vi "RT Loop - Acquisition and Logging V2.vi"(8 "error in (no error)":errorcluster, 9 "Acquisition and Logging Configuration":T1={"Data Rate"=1, "Samples per Read"=0, "Number of Reads to Save"=0, "Data File Name"="", "TDMS Properties"=[], "Number of Channels"=4, "Channel Scale Array"=[0.0, 0.0, 0.0, 0.0, 1.0, 1.0, 1.0, 1.0], "Channel Names"=[], "Trigger - RMS Value"=0.0, "Trigger - Channel"=0, "Trigger - Time (Minute)"=0} {"Data Rate" items=["51.200 kS/s (NI 9234)"=1, "25.600 kS/s (NI 9234)"=2, "17.067 kS/s (NI 9234)"=3, "12.800 kS/s (NI 9234)"=4, "10.240 kS/s (NI 9234)"=5, "8.533 kS/s (NI 9234)"=6, "7.314 kS/s (NI 9234)"=7, "6.400 kS/s (NI 9234)"=8, "5.689 kS/s (NI 9234)"=9, "5.120 kS/s (NI 9234)"=10, "4.654 kS/s (NI 9234)"=11, "4.267 kS/s (NI 9234)"=12, "3.938 kS/s (NI 9234)"=13, "3.657 kS/s (NI 9234)"=14, "3.413 kS/s (NI 9234)"=15, "3.200 kS/s (NI 9234)"=16, "3.012 kS/s (NI 9234)"=17, "2.845 kS/s (NI 9234)"=18, "2.695 kS/s (NI 9234)"=19, "2.560 kS/s (NI 9234)"=20, "2.438 kS/s (NI 9234)"=21, "2.328 kS/s (NI 9234)"=22, "2.226 kS/s (NI 9234)"=23, "2.133 kS/s (NI 9234)"=24, "2.048 kS/s (NI 9234)"=25, "1.969 kS/s (NI 9234)"=26, "1.896 kS/s (NI 9234)"=27, "1.829 kS/s (NI 9234)"=28, "1.765 kS/s (NI 9234)"=29, "1.707 kS/s (NI 9234)"=30, "1.652 kS/s (NI 9234)"=31]}, 10 "Acquisition and Logging Queue":refnum<queue>, 11 "Message Queue":refnum<queue>) -> ()   [LabVIEW 2015]
uses:
  controls/FPGA VI Reference.ctl
  support/Message Queue/Message Queue.lvlib
  Globals/Global - Configuration Options.vi
  Globals/Global - Monitoring Variables.vi
  support/Message Queue/Message Cluster.ctl
  controls/Acquisition and Logging Configuration.ctl
  <vilib>/LabVIEW Targets/FPGA/cRIO/shared/nicrio_ModuleControls/nicrio_cRIO-9234_DataRatesRing2.ctl
  controls/TDMS Properties.ctl
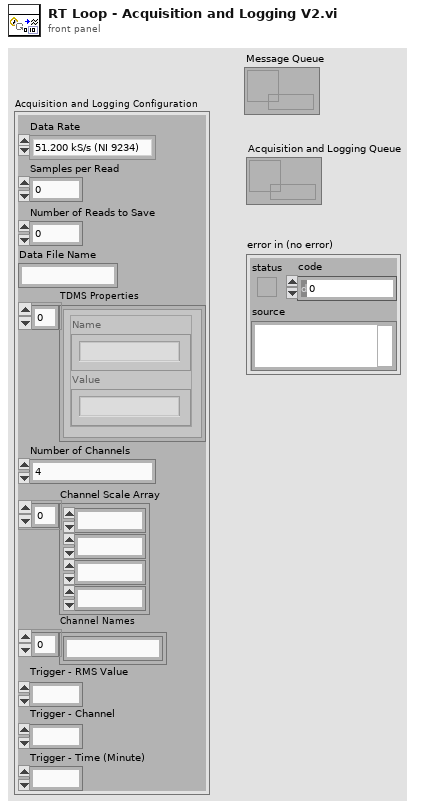
[diagram p1: front panel]
types:
  T1 = typedef "Acquisition and Logging Configuration.ctl" = cluster{"Data Rate":T2, "Samples per Read":i32, "Number of Reads to Save":i32, "Data File Name":string, "TDMS Properties":T3[], "Number of Channels":i32, "Channel Scale Array":fxp<+,24,12>[], "Channel Names":string[], "Trigger - RMS Value":dbl, "Trigger - Channel":i32, "Trigger - Time (Minute)":i32}
  T2 = typedef "nicrio_cRIO-9234_DataRatesRing2.ctl" = u8
  T3 = typedef "TDMS Properties.ctl" = cluster{"Name":string, "Value":string}
  T4 = typedef "FPGA VI Reference.ctl" = refnum<k20>
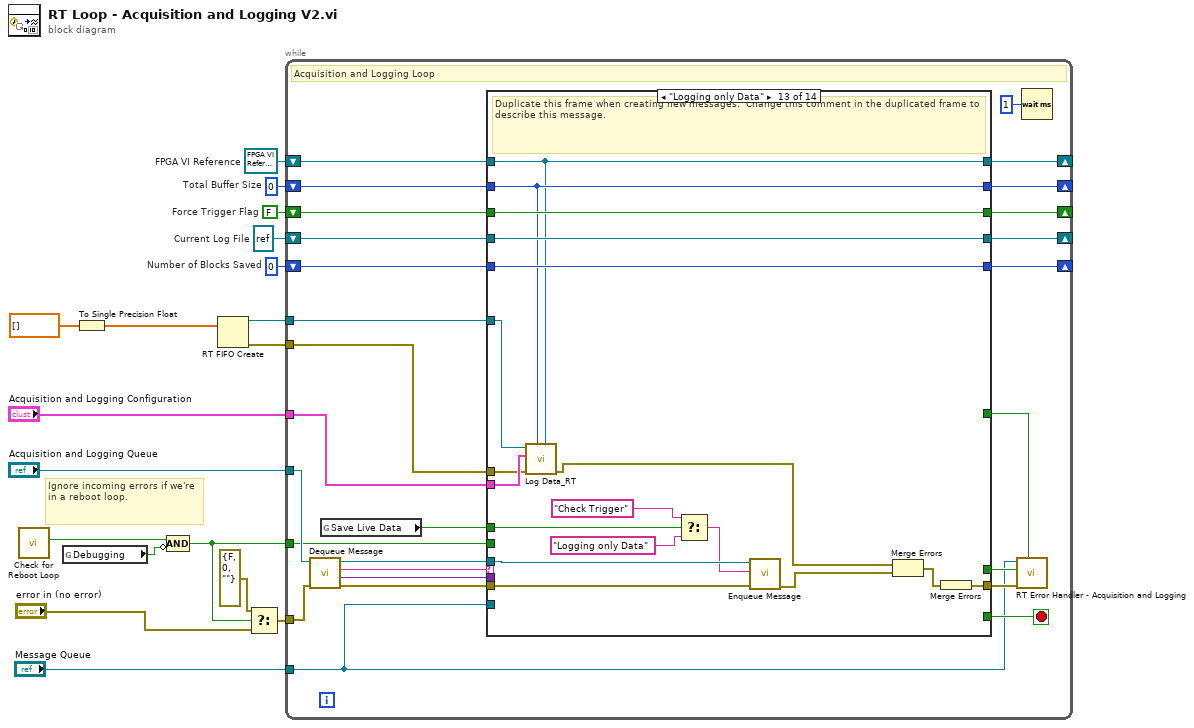
[diagram p0: block diagram]
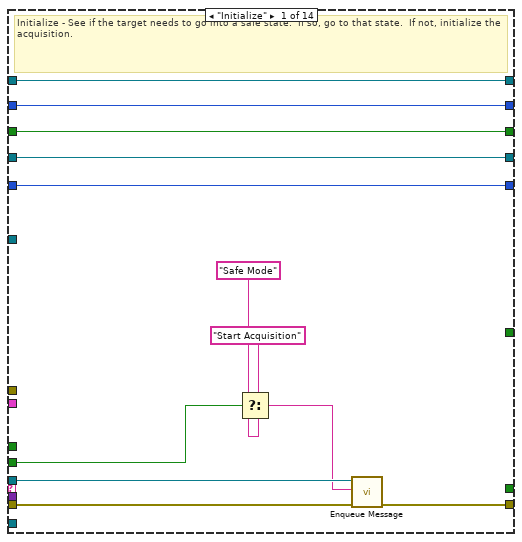
[diagram p2: hidden frame]
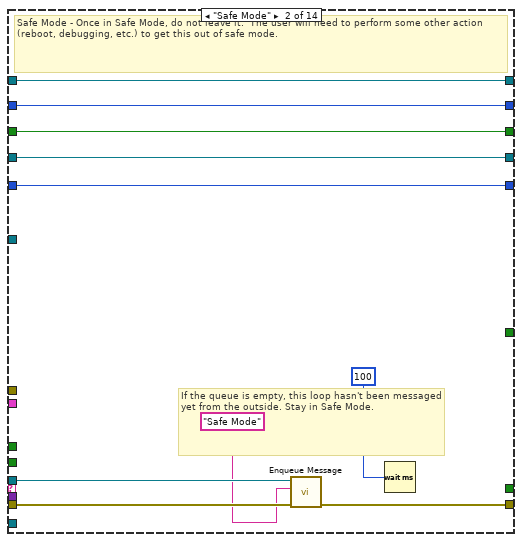
[diagram p3: hidden frame]
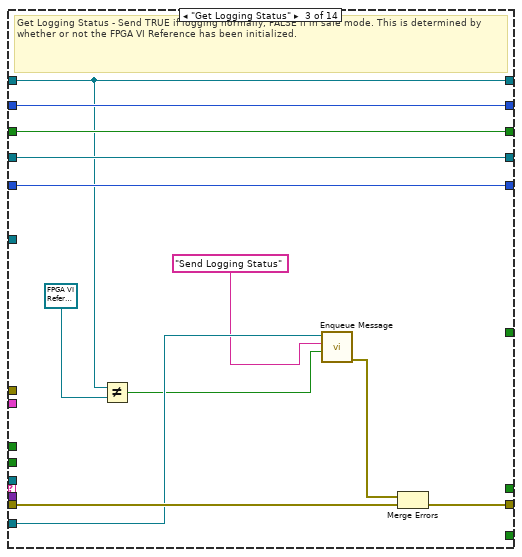
[diagram p4: hidden frame]
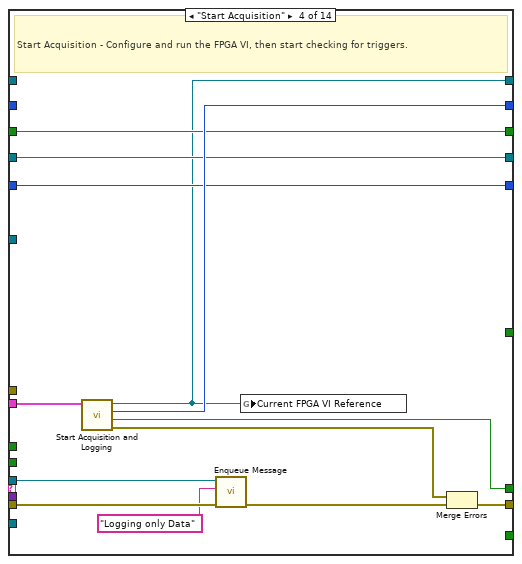
[diagram p5: hidden frame]
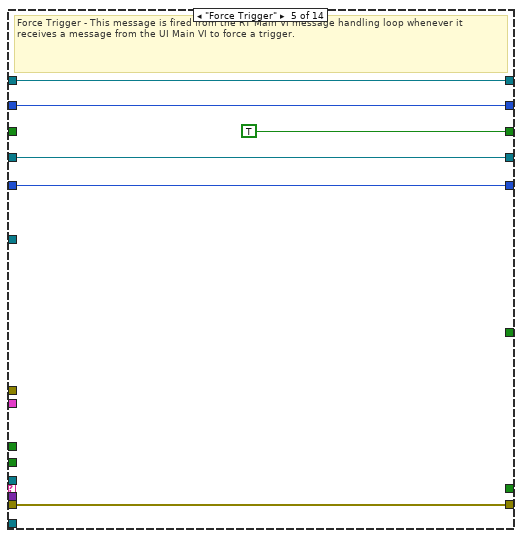
[diagram p6: hidden frame]
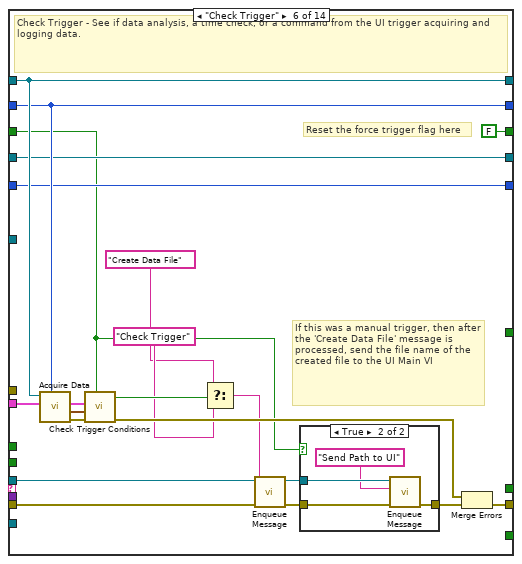
[diagram p7: hidden frame]
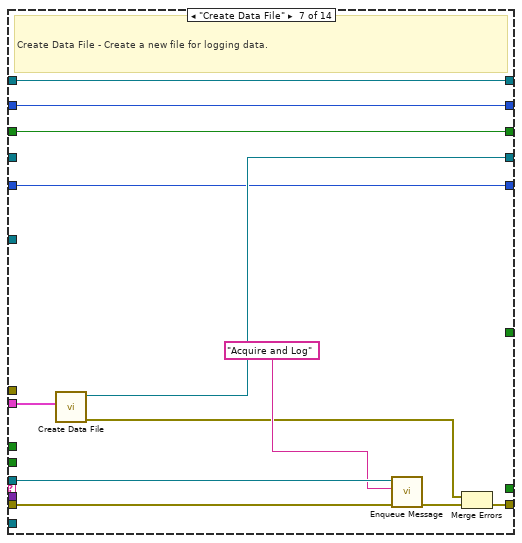
[diagram p9: hidden frame]
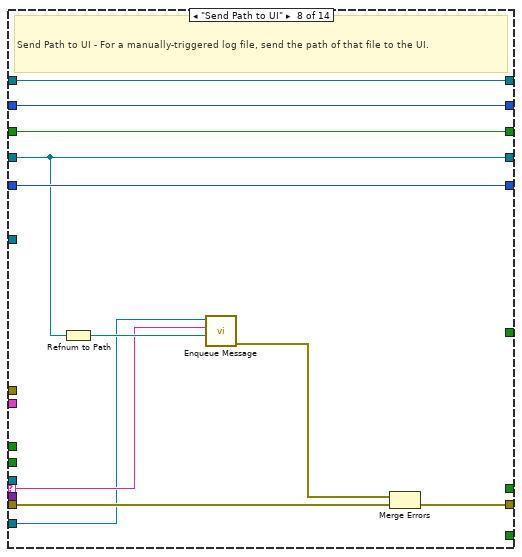
[diagram p10: hidden frame]
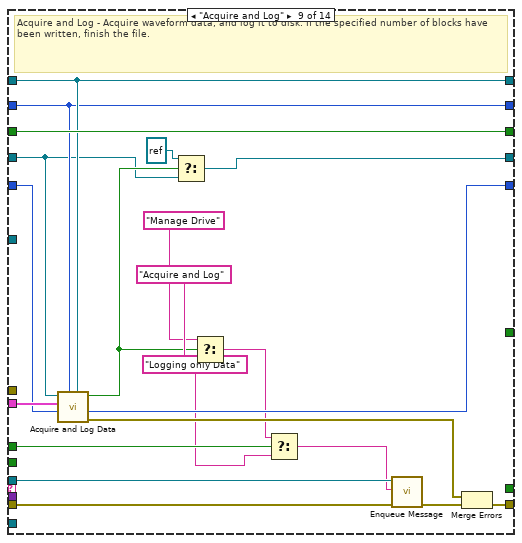
[diagram p11: hidden frame]
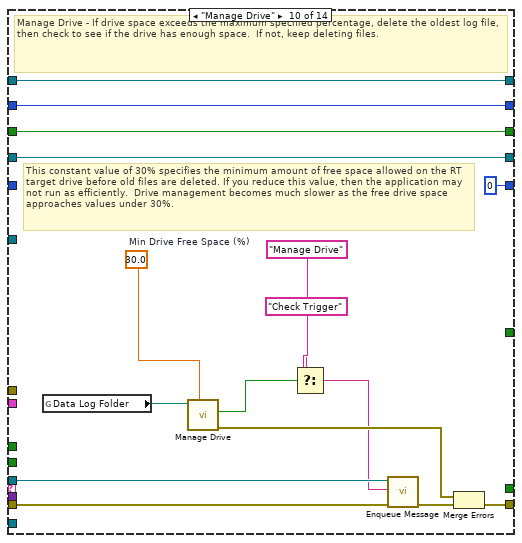
[diagram p12: hidden frame]
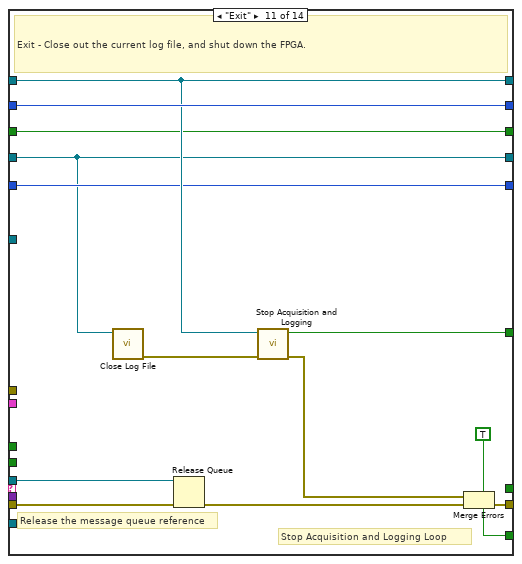
[diagram p13: hidden frame]
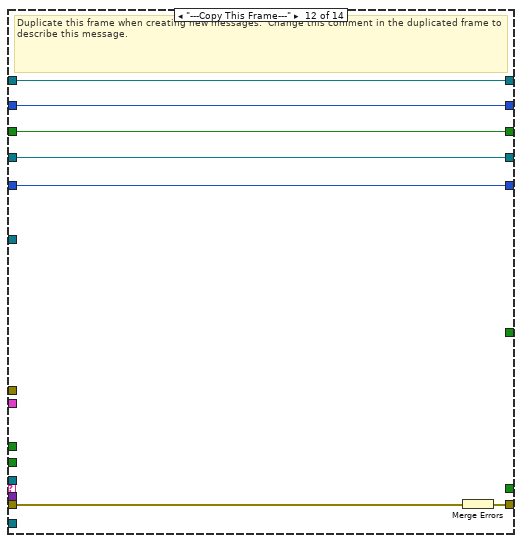
[diagram p14: hidden frame]
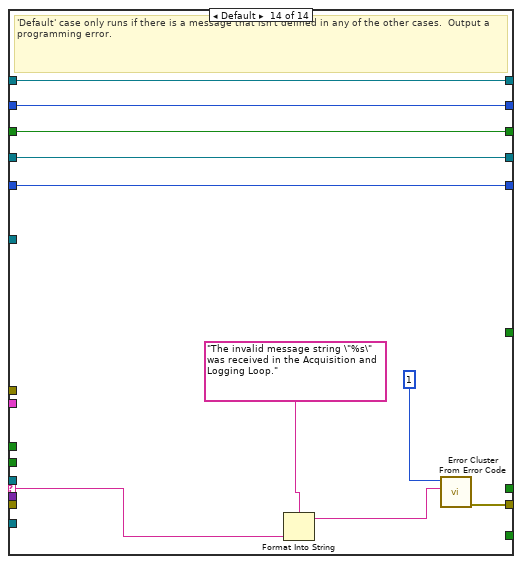
[diagram p15: hidden frame]
diagram:
  w11 = 0  # Number of Blocks Saved
  w12 = refnum<k34> refnum  # Current Log File
  w13 = FALSE  # Force Trigger Flag
  w15 = 0  # Total Buffer Size
  w16 = T4 refnum  # FPGA VI Reference
  # "Ignore incoming errors if we're in a reboot loop."
  n1 = call "Check for Reboot Loop.vi"() -> ("Start in Safe Mode?"=w7:bool)  [unwired: 10 in, 1 out]
  n2 = global read "Global - Configuration Options.vi" "Debugging"() -> (w6:bool)
  n3 = To Single Precision Float(number=dbl[] []) -> (single precision float=w3:sgl[])
  n4 = Compound Arithmetic op=AND(w7, invert w6) -> (w5:bool)
  n5 = RT FIFO Create(1:w3) -> (8:w4:refnum<k33>, 11:w1:errorcluster)  [unwired: 7 in, 1 out]
  n6 = Select(t=errorcluster {"status"=FALSE, "code"=0, "source"=""}, s=w5, f="error in (no error)") -> (s? t:f=w9:errorcluster)
  n7 = while {
    tunnel: "Acquisition and Logging Queue" -> [w41]
    tunnel: "Message Queue" -> [w25]
    shift-right: [w36] -> _
    shift-left: w16 -> [w38]
    shift-right: [w35] -> _
    shift-left: w15 -> [w37]
    tunnel: "Acquisition and Logging Configuration" -> [w34]
    shift-right: [w30] -> _
    shift-left: w13 -> [w31]
    shift-right: [w28] -> _
    shift-left: w12 -> [w29]
    shift-right: [w26] -> _
    shift-left: w11 -> [w27]
    tunnel: w9 -> [w23]
    tunnel: w5 -> [w22]
    tunnel: w4 -> [w20]
    tunnel: w1 -> [w19]
    stop <- w45 stop-if-true
    # "Acquisition and Logging Loop"
    n8 = call "Dequeue Message.vi"("error in (no error)"=w23, "Message Queue"=w41) -> ("error out"=w44:errorcluster, "Message Data"=w42:variant, "Message"=w43:string, "dup Message Queue"=w39:refnum<queue>)  [unwired: 6 in]
    n9 = global read "Global - Monitoring Variables.vi" "Save Live Data"() -> (w21:bool)
    n10 = case "Message Cases" shown="\"Logging only Data\"" w43 {
      selector: w43 -> [_ _ _ _ _ _ _ w140 _ _ _ _ _ w231]
      tunnel: w39 -> [w54 w64 _ w85 _ w110 w131 _ w165 w177 w197 _ w218 _]
      tunnel: w44 -> [w55 w65 w79 w92 w98 w118 w135 w147 w168 w184 w193 w204 w215 _]
      tunnel: [w47 w63 w71 w90 w98 w117 w134 w138 w167 w180 w194 w203 w222 w229] -> w40
      tunnel: [_ _ _ _ _ _ _ _ _ _ TRUE _ _ _] -> w45
      tunnel: w42 -> [_ _ _ _ _ _ _ _ _ _ _ _ _ _]
      tunnel: w38 -> [w57 w67 w74 _ w97 w119 w136 w146 w159 w183 w191 w202 w208 w227]
      tunnel: w37 -> [w56 w66 w78 _ w96 w115 w133 w145 w158 w182 w192 w201 w209 w226]
      tunnel: [w57 w67 w74 w80 w97 w119 w136 w146 w159 w183 w191 w202 w208 w227] -> w36
      tunnel: [w56 w66 w78 w87 w96 w115 w133 w145 w158 w182 w192 w201 w209 w226] -> w35
      tunnel: w34 -> [_ _ _ w91 _ w116 w128 _ w163 _ _ _ w210 _]
      tunnel: [_ _ _ w88 _ _ _ _ _ _ _ _ _ _] -> w32
      tunnel: w31 -> [w50 w62 w77 w83 _ w99 w129 w144 w164 w170 w189 w200 w221 w225]
      tunnel: [w50 w62 w77 w83 TRUE ("Force Trigger Flag") FALSE ("Force Trigger Flag") w129 w144 w164 w170 w189 w200 w221 w225] -> w30
      tunnel: w29 -> [w49 w61 w76 w82 w95 w105 _ w142 w154 w181 w186 w199 w220 w224]
      tunnel: [w49 w61 w76 w82 w95 w105 w126 w142 w153 w181 w186 w199 w220 w224] -> w28
      tunnel: w27 -> [w48 w60 w75 w81 w93 w104 w125 w143 w157 _ w188 w198 w219 w223]
      tunnel: [w48 w60 w75 w81 w93 w104 w125 w143 w156 0 ("Number of Blocks Saved") w188 w198 w219 w223] -> w26
      tunnel: w25 -> [_ _ w72 _ _ _ _ w139 _ _ _ _ _ _]
      tunnel: [_ _ _ _ _ _ _ _ _ _ w185 _ _ _] -> w24
      tunnel: w22 -> [w46 _ _ _ _ _ _ _ _ _ _ _ _ _]
      tunnel: w21 -> [_ _ _ _ _ _ _ _ w151 _ _ _ w212 _]
      tunnel: w20 -> [_ _ _ _ _ _ _ _ _ _ _ _ w206 _]
      tunnel: w19 -> [_ _ _ _ _ _ _ _ _ _ _ _ w205 _]
      frame "Initialize" {
        # "Initialize - See if the target needs to go into a safe state.  If so, go to that state.  If not, initialize the acquisition."
        n11 = Select(t="Safe Mode", s=w46, f="Start Acquisition") -> (s? t:f=w51:string)
        n12 = call "Enqueue Message.vi"("error in (no error)"=w55, "Message"=w51, "Message Queue"=w54) -> ("error out"=w47:errorcluster)  [unwired: 7 in, 1 out]
      }
      frame "Safe Mode" {
        # "If the queue is empty, this loop hasn't been messaged yet from the outside. Stay in Safe Mode."
        # "Safe Mode - Once in Safe Mode, do not leave it.  The user will need to perform some other action (reboot, debugging, etc.) to get this out of safe mode."
        n13 = call "Enqueue Message.vi"("error in (no error)"=w65, "Message"="Safe Mode", "Message Queue"=w64) -> ("error out"=w63:errorcluster)  [unwired: 7 in, 1 out]
        n14 = Wait (ms)(milliseconds to wait=u32 100) -> ()  [unwired: 1 out]
      }
      frame "Get Logging Status" {
        # "Get Logging Status - Send TRUE if logging normally, FALSE if in safe mode. This is determined by whether or not the FPGA VI Reference has been initialized."
        n15 = Not Equal?(x=w74, y=T4 refnum ("FPGA VI Reference")) -> (x != y?=w69:bool)
        n16 = call "Enqueue Message.vi"("Message Data"=w69, "Message"="Send Logging Status", "Message Queue"=w72) -> ("error out"=w70:errorcluster)  [unwired: 7 in, 1 out]
        n17 = Merge Errors(w70, w79) -> (w71:errorcluster)
      }
      frame "Start Acquisition" {
        # "Start Acquisition - Configure and run the FPGA VI, then start checking for triggers."
        n18 = call "Start Acquisition and Logging.vi"("Acquisition and Logging Configuration"=w91) -> ("error out"=w89:errorcluster, "Wait on IRQ Timeout?"=w88:bool, "Total Buffer Size"=w87:i32, "FPGA VI Reference Out"=w80:T4)  [unwired: 7 in]
        n19 = call "Enqueue Message.vi"("error in (no error)"=w92, "Message"="Logging only Data", "Message Queue"=w85) -> ("error out"=w86:errorcluster)  [unwired: 7 in, 1 out]
        n20 = global write "Global - Monitoring Variables.vi" "Current FPGA VI Reference"(w80) -> ()
        n21 = Merge Errors(w89, w86) -> (w90:errorcluster)
      }
      frame "Force Trigger" {
        # "Force Trigger - This message is fired from the RT Main VI message handling loop whenever it receives a message from the UI Main VI to force a trigger."
      }
      frame "Check Trigger" {
        # "If this was a manual trigger, then after the 'Create Data File' message is processed, send the file name of the created file to the UI Main VI"
        # "Reset the force trigger flag here"
        # "Check Trigger - See if data analysis, a time check, or a command from the UI trigger acquiring and logging data."
        n22 = call "Acquire Data.vi"("Total Buffer Size"=w115, "Acquisition and Logging Configuration"=w116, "FPGA VI Reference"=w119) -> ("error out"=w113:errorcluster, "Waveform Data"=w112:waveform(sgl)[], "dup Acquisition and Logging Configuration"=w111:T1)  [unwired: 6 in]
        n23 = call "Check Trigger Conditions.vi"("Force Trigger?"=w99, "error in (no error)"=w113, "Waveform Data"=w112, "Acquisition and Logging Configuration"=w111) -> ("error out"=w114:errorcluster, "Trigger Condition Met?"=w109:bool)  [unwired: 6 in]
        n24 = Select(t="Create Data File", s=w109, f="Check Trigger") -> (s? t:f=w106:string)
        n25 = call "Enqueue Message.vi"("error in (no error)"=w118, "Message"=w106, "Message Queue"=w110) -> ("error out"=w102:errorcluster, "dup Message Queue"=w100:refnum<queue>)  [unwired: 7 in]
        n26 = case shown="True" w99 {
          tunnel: w102 -> [w120 w123]
          tunnel: [w120 w124] -> w101
          tunnel: w100 -> [_ w122]
          frame False {
          }
          frame True {
            n27 = call "Enqueue Message.vi"("error in (no error)"=w123, "Message"="Send Path to UI", "Message Queue"=w122) -> ("error out"=w124:errorcluster)  [unwired: 7 in, 1 out]
          }
        }
        n28 = Merge Errors(w114, w101) -> (w117:errorcluster)
      }
      frame "Create Data File" {
        # "Create Data File - Create a new file for logging data."
        n29 = call "Create Data File.vi"("Acquisition and Logging Configuration"=w128) -> ("error out"=w127:errorcluster, "TDMS File Reference"=w126:refnum<k34>)  [unwired: 9 in]
        n30 = call "Enqueue Message.vi"("error in (no error)"=w135, "Message"="Acquire and Log", "Message Queue"=w131) -> ("error out"=w132:errorcluster)  [unwired: 7 in, 1 out]
        n31 = Merge Errors(w127, w132) -> (w134:errorcluster)
      }
      frame "Send Path to UI" {
        # "Send Path to UI - For a manually-triggered log file, send the path of that file to the UI."
        n32 = Refnum to Path(1:w142) -> (0:w141:path)
        n33 = call "Enqueue Message.vi"("Message Data"=w141, "Message"=w140, "Message Queue"=w139) -> ("error out"=w137:errorcluster)  [unwired: 7 in, 1 out]
        n34 = Merge Errors(w137, w147) -> (w138:errorcluster)
      }
      frame "Acquire and Log" {
        # "Acquire and Log - Acquire waveform data, and log it to disk. If the specified number of blocks have been written, finish the file."
        n35 = call "Acquire and Log Data.vi"("FPGA VI Reference"=w159, "Total Buffer Size"=w158, "Number of Blocks Saved in"=w157, "Acquisition and Logging Configuration"=w163, "TDMS File Reference"=w154) -> ("error out"=w162:errorcluster, "Number of Blocks Saved out"=w156:i32, "Logging Complete?"=w155:bool)  [unwired: 4 in]
        n36 = Select(t=refnum<k34> refnum, s=w155, f=w154) -> (s? t:f=w153:refnum<k34>)
        n37 = Select(t="Manage Drive", s=w155, f="Acquire and Log") -> (s? t:f=w149:string)
        n38 = Select(t=w149, s=w151, f="Logging only Data") -> (s? t:f=w148:string)
        n39 = call "Enqueue Message.vi"("error in (no error)"=w168, "Message"=w148, "Message Queue"=w165) -> ("error out"=w166:errorcluster)  [unwired: 7 in, 1 out]
        n40 = Merge Errors(w162, w166) -> (w167:errorcluster)
      }
      frame "Manage Drive" {
        w179 = 30.0  # Min Drive Free Space (%)
        # "This constant value of 30% specifies the minimum amount of free space allowed on the RT target drive before old files are deleted. If you reduce this value, then the application may not run as efficiently.  Drive management becomes much slower as the free drive space approaches values under 30%."
        # "Manage Drive - If drive space exceeds the maximum specified percentage, delete the oldest log file, then check to see if the drive has enough space.  If not, keep deleting files."
        n41 = global read "Global - Configuration Options.vi" "Data Log Folder"() -> (w169:path)
        n42 = call "Manage Drive.vi"("Min Drive Free Space (%)"=w179, "Data Folder"=w169) -> ("error out"=w176:errorcluster, "Drive Space Below Limit"=w175:bool)  [unwired: 8 in]
        n43 = Select(t="Manage Drive", s=w175, f="Check Trigger") -> (s? t:f=w172:string)
        n44 = call "Enqueue Message.vi"("error in (no error)"=w184, "Message"=w172, "Message Queue"=w177) -> ("error out"=w178:errorcluster)  [unwired: 7 in, 1 out]
        n45 = Merge Errors(w176, w178) -> (w180:errorcluster)
      }
      frame "Exit" {
        # "Stop Acquisition and Logging Loop"
        # "Release the message queue reference"
        # "Exit - Close out the current log file, and shut down the FPGA."
        n46 = call "Close Log File.vi"("Log File"=w186) -> ("error out"=w187:errorcluster)  [unwired: 10 in]
        n47 = Release Queue(queue=w197, error in (no error)=w193) -> (error out=w195:errorcluster)  [unwired: 1 in, 2 out]
        n48 = call "Stop Acquisition and Logging.vi"("error in (no error)"=w187, "FPGA VI Reference"=w191) -> ("error out"=w190:errorcluster, "Stop FPGA Timeout?"=w185:bool)  [unwired: 8 in]
        n49 = Merge Errors(w190, w195) -> (w194:errorcluster)
      }
      frame "---Copy This Frame---" {
        # "Duplicate this frame when creating new messages.  Change this comment in the duplicated frame to describe this message."
        n50 = Merge Errors(w204) -> (w203:errorcluster)
      }
      frame "Logging only Data" {
        # "Duplicate this frame when creating new messages.  Change this comment in the duplicated frame to describe this message."
        n51 = call "Log Data_RT.vi"("FPGA VI Reference"=w208, "Total Buffer Size"=w209, "error in (no error)"=w205, "Acquisition and Logging Configuration"=w210, "rt fifo"=w206) -> ("error out"=w207:errorcluster)  [unwired: 6 in]
        n52 = Select(t="Check Trigger" ("Message"), s=w212, f="Logging only Data" ("Message")) -> (s? t:f=w213:string)
        n53 = call "Enqueue Message.vi"("error in (no error)"=w215, "Message"=w213, "Message Queue"=w218) -> ("error out"=w217:errorcluster)  [unwired: 7 in, 1 out]
        n54 = Merge Errors(w207, w217) -> (w216:errorcluster)
        n55 = Merge Errors(w216) -> (w222:errorcluster)
      }
      frame Default {
        # "'Default' case only runs if there is a message that isn't defined in any of the other cases.  Output a programming error."
        n56 = Format Into String(format string="The invalid message string \"%s\" was received in the Acquisition and Logging Loop." ("Unknown Message Error Text"), w231) -> (resulting string=w228:string)  [unwired: 2 in, 1 out]
        n57 = call <vilib>:"Error Cluster From Error Code.vi"("error message (\"\")"=w228, "error code (0)"=1) -> ("error out"=w229:errorcluster)  [unwired: 7 in]
      }
    }
    n58 = call "RT Error Handler - Acquisition and Logging.vi"("Stop FPGA Timeout"=w24, "error in (no error)"=w40, "IRQ Timeout"=w32, "Message Queue"=w25) -> ()  [unwired: 7 in, 1 out]
    n59 = Wait (ms)(milliseconds to wait=u32 1) -> ()  [unwired: 1 out]
  }
